vi "(SubVI)Ex and Force.vi"(3 "control Cluster":T2={"laser power (mW)"=10.0, "center position shift (um)"=0.0001, "center QPD shift (V)"=0.0001, "Fc-cal-array"=[0.004414, 0.00367], "Convf-cal-array"=[0.19240621, 0.01244886], "Length offset"=400.0, "Force offset"=4.0, "trap height(nm)"=300.0, "bead radius(nm)"=515.0, "xDNA cut outside (nm)"=2000.0, "initial parameters"=[40.0, 1150.0], "fit only one side?"=FALSE, "T=positive (RHS)\nF=negative (LHS)"=FALSE, "Position Array Out"=[], "QPD signal Out"=[], "ci"=0.0, "yi"=0.0, "cr"=0.0, "yr"=0.0, "Force constant (pN/nm)"=0.0154, "conversion factor (V/um)"=2.6, "best fit parameters"=[], "best nonlinear fit"=[], "residue"=0.0, "Force-cut 2"=[], "xDNA-cut 2"=[]}) -> (0 "indicator Cluster":T1, 1 "Force-cut":dbl[](array[numeric]), 2 "xDNA-cut":dbl[](array[numeric]))   [LabVIEW 2014]
uses:
  Control cluster.ctl
panel:
  # "Lp"
  # "L0"
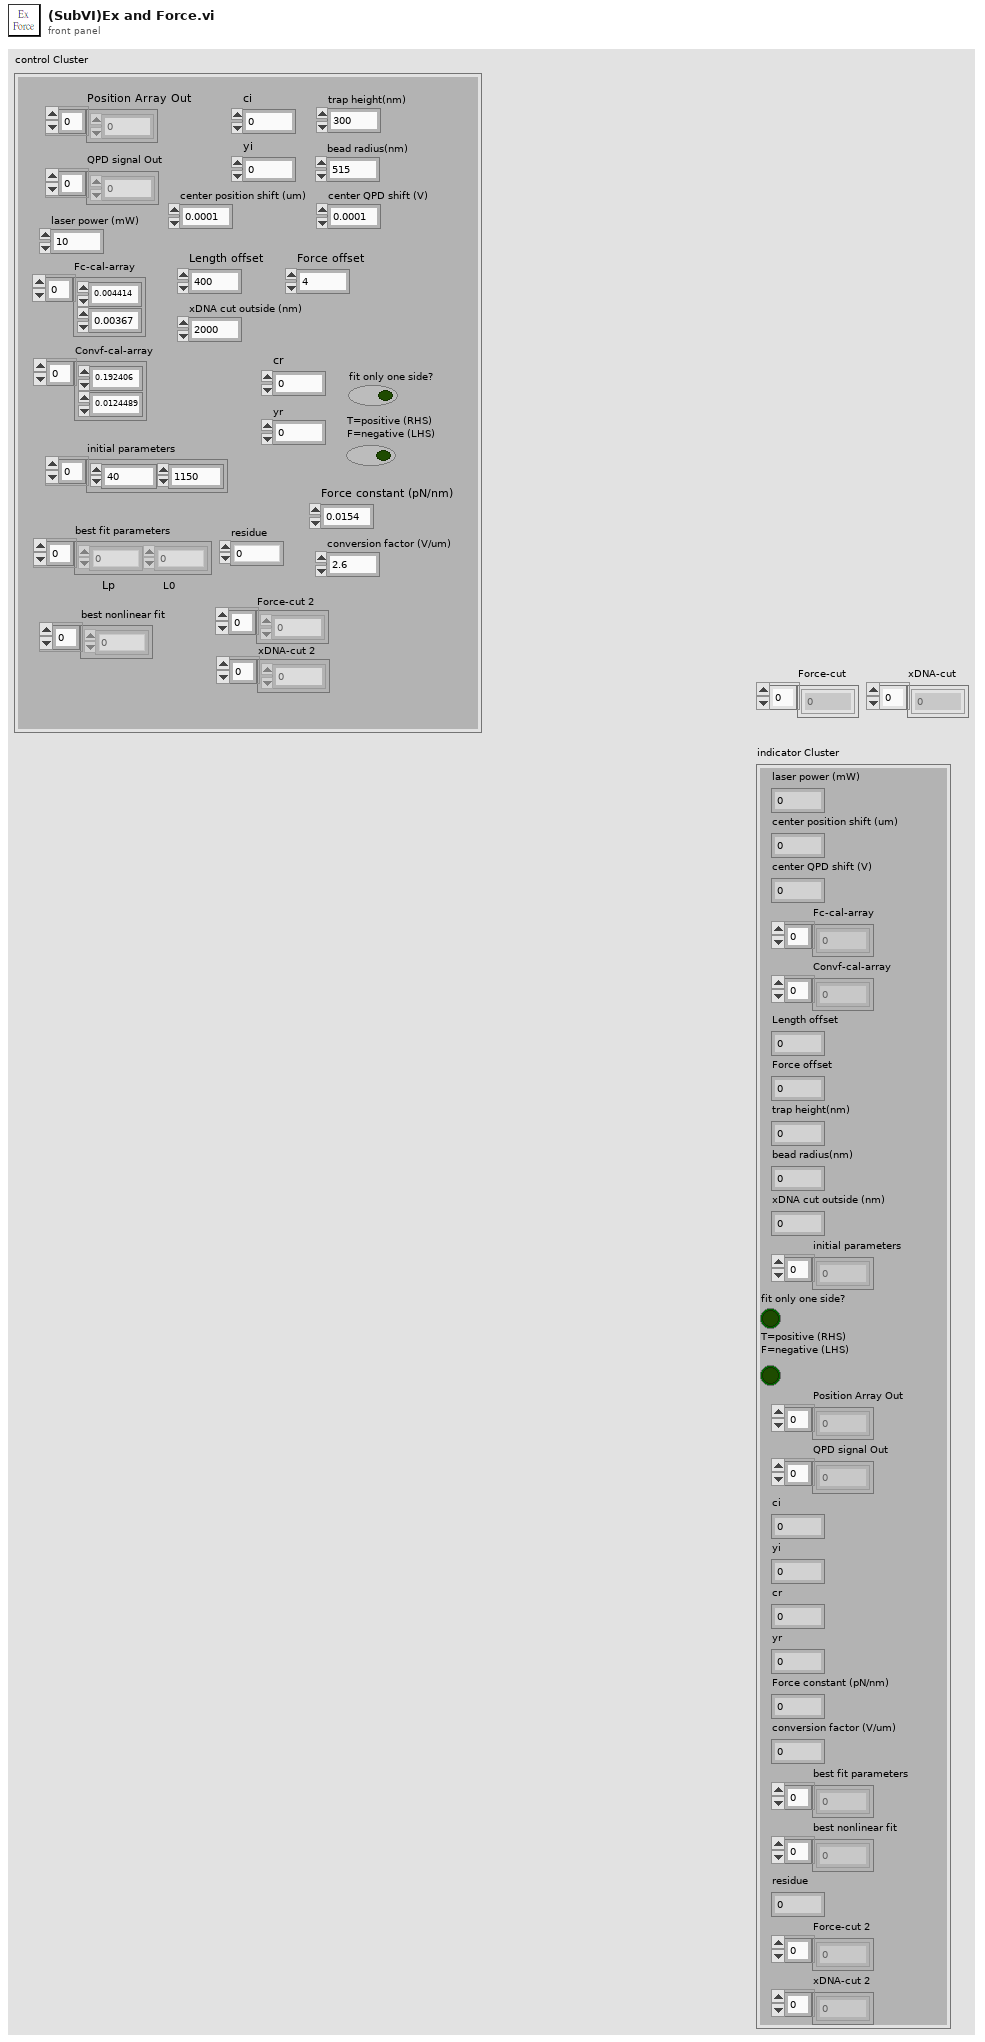
[diagram p1: front panel]
types:
  T1 = cluster{"laser power (mW)":dbl, "center position shift (um)":dbl, "center QPD shift (V)":dbl, "Fc-cal-array":dbl[], "Convf-cal-array":dbl[], "Length offset":dbl, "Force offset":dbl, "trap height(nm)":dbl, "bead radius(nm)":dbl, "xDNA cut outside (nm)":dbl, "initial parameters":dbl[], "fit only one side?":bool, "T=positive (RHS)\nF=negative (LHS)":bool, "Position Array Out":dbl[], "QPD signal Out":dbl[], "ci":dbl, "yi":dbl, "cr":dbl, "yr":dbl, "Force constant (pN/nm)":dbl, "conversion factor (V/um)":dbl, "best fit parameters":dbl[], "best nonlinear fit":dbl[], "residue":dbl, "Force-cut 2":dbl[], "xDNA-cut 2":dbl[]}
  T2 = typedef "Control cluster.ctl" = cluster{"laser power (mW)":dbl, "center position shift (um)":dbl, "center QPD shift (V)":dbl, "Fc-cal-array":dbl[], "Convf-cal-array":dbl[], "Length offset":dbl, "Force offset":dbl, "trap height(nm)":dbl, "bead radius(nm)":dbl, "xDNA cut outside (nm)":dbl, "initial parameters":dbl[], "fit only one side?":bool, "T=positive (RHS)\nF=negative (LHS)":bool, "Position Array Out":dbl[], "QPD signal Out":dbl[], "ci":dbl, "yi":dbl, "cr":dbl, "yr":dbl, "Force constant (pN/nm)":dbl, "conversion factor (V/um)":dbl, "best fit parameters":dbl[], "best nonlinear fit":dbl[], "residue":dbl, "Force-cut 2":dbl[], "xDNA-cut 2":dbl[]}
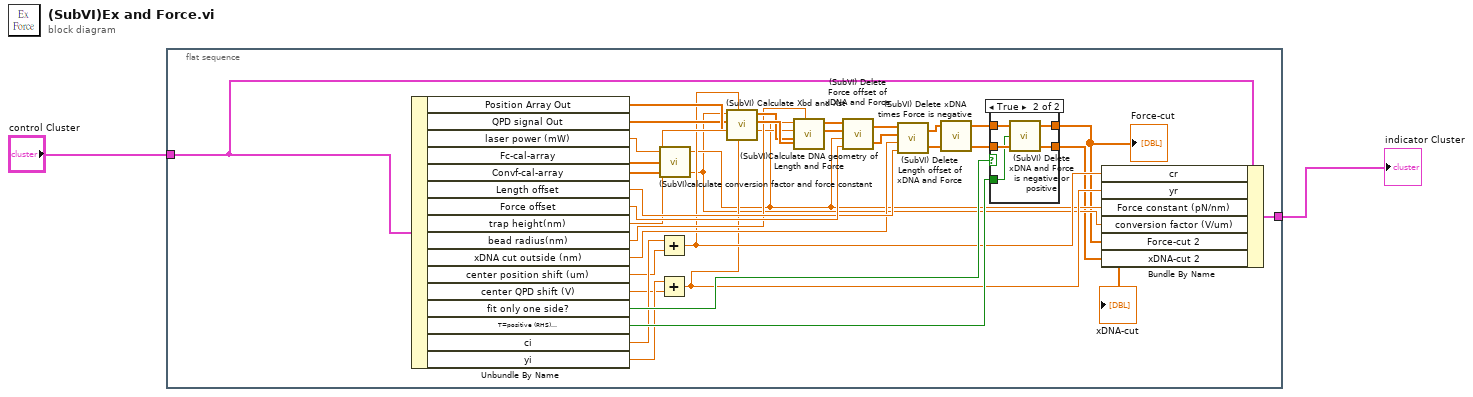
[diagram p0: block diagram]
diagram:
  n1 = flat-sequence {
    tunnel: [w4] -> w2
    tunnel: "control Cluster" -> [w3]
    frame #0 {
      n2 = Unbundle By Name(w3) -> ("Position Array Out"=w18:dbl[], "QPD signal Out"=w17:dbl[], "laser power (mW)"=w28:dbl, "Fc-cal-array"=w27:dbl[], "Convf-cal-array"=w26:dbl[], "Length offset"=w24:dbl, "Force offset"=w25:dbl, "trap height(nm)"=w21:dbl, "bead radius(nm)"=w22:dbl, "xDNA cut outside (nm)"=w23:dbl, "center position shift (um)"=w14:dbl, "center QPD shift (V)"=w13:dbl, "fit only one side?"=w20:bool, "T=positive (RHS)\nF=negative (LHS)"=w19:bool, "ci"=w16:dbl, "yi"=w15:dbl)
      n3 = Add(x=w16, y=w14) -> (x+y=w12:dbl)
      n4 = Add(x=w15, y=w13) -> (x+y=w11:dbl)
      n5 = call "(SubVI)calculate conversion factor and force constant.vi"("X=T\nY=F"=w26, 4:w27, "laser power (mW)"=w28) -> ("conversion factor (V/um)"=w9:dbl, "force constant (pN/nm)"=w10:dbl)  [unwired: 1 in]
      n6 = call "(SubVI) Calculate Xbd and Xst.vi"("yr"=w11, "cr"=w12, "Stage Position"=w18, "QPD signal"=w17, "conversion factor (V/um)"=w9) -> ("Xst"=w36:dbl[], "Xbd"=w35:dbl[])  [unwired: 5 in]
      n7 = call "(SubVI)Calculate DNA geometry of Length and Force.vi"("trap height(nm)"=w36, "bead radius(nm)"=w22, 9:w35, "Xst"=w21, "Xbd"=w10) -> ("xDNA"=w34:dbl[], "Force"=w33:dbl[])  [unwired: 4 in, 1 out]
      n8 = call "(SubVI) Delete Force offset of xDNA and Force.vi"("Force offset"=w25, "force constant"=w10, "xDNA"=w34, "Force"=w33) -> ("cut-full xDNA"=w31:dbl[], "cut-full Force"=w32:dbl[])
      n9 = call "(SubVI) Delete Length offset of xDNA and Force.vi"("Length offset"=w24, "xDNA cut outside (nm)"=w23, "xDNA"=w31, "Force"=w32) -> ("cut-full xDNA"=w29:dbl[], "cut-full Force"=w30:dbl[])
      n10 = call "(SubVI) Delete xDNA times Force is negative.vi"("xDNA"=w29, "Force"=w30) -> ("xDNA-cut"=w7:dbl[], "Force-cut"=w8:dbl[])  [unwired: 2 in]
      n11 = case shown="True" w20 {
        tunnel: w8 -> [w38 w43]
        tunnel: w7 -> [w37 w42]
        tunnel: [w37 w41] -> w6
        tunnel: [w38 w40] -> w5
        tunnel: w19 -> [_ w39]
        frame False {
        }
        frame True {
          n12 = call "(SubVI) Delete xDNA and Force is negative or positive.vi"("xDNA"=w42, "T=positive (RHS)\nF=negative (LHS)"=w39, "Force"=w43) -> ("xDNA-cut"=w41:dbl[], "Force-cut"=w40:dbl[])  [unwired: 1 in]
        }
      }
      "Force-cut" <- w5
      "xDNA-cut" <- w6
      n13 = Bundle By Name(cluster=w3, "cr"=w12, "yr"=w11, "Force constant (pN/nm)"=w10, "conversion factor (V/um)"=w9, "Force-cut 2"=w5, "xDNA-cut 2"=w6) -> (w4:T2)
    }
  }
  "indicator Cluster" <- w2
